vi "IdentifierResult.vi"(8 "error in (no error)":errorcluster, 11 "map":map{string, string}(c390)) -> (0 "error out":errorcluster, 2 "status":string, 3 "description":string)   [LabVIEW 2021]
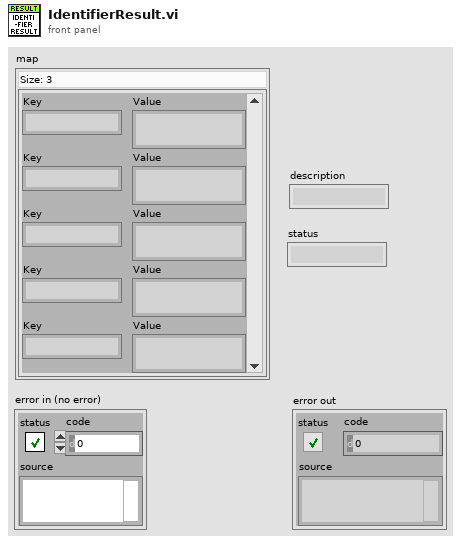
[diagram p1: front panel]
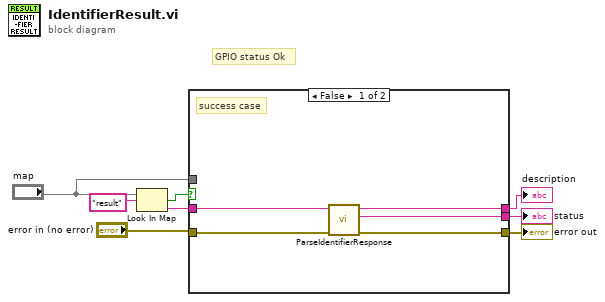
[diagram p0: block diagram]
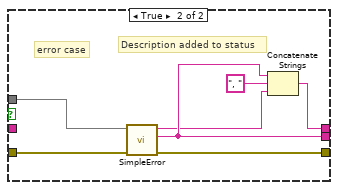
[diagram p2: hidden frame]
diagram:
  # "GPIO status Ok"
  n1 = Look In Map(map="map", key="result") -> (key not found?=w6:bool, value=w7:string)  [unwired: 1 in]
  n2 = case shown="False" w6 {
    tunnel: w7 -> [w13 _]
    tunnel: "error in (no error)" -> [w12 w20]
    tunnel: [w11 w19] -> w4
    tunnel: "map" -> [_ w18]
    tunnel: [w9 w14] -> w1
    tunnel: [w10 w16] -> w2
    frame False {
      # "success case"
      n3 = call "ParseIdentifierResponse.vi"("error in (no error)"=w12, "Value"=w13) -> ("error out"=w11:errorcluster, "status"=w10:string, "description"=w9:string)  [unwired: 7 in]
    }
    frame True {
      # "Description added to status"
      # "error case"
      n4 = call "SimpleError.vi"("error in (no error)"=w20, "map"=w18) -> ("error out"=w19:errorcluster, "status"=w16:string, "description"=w15:string)  [unwired: 7 in]
      n5 = Concatenate Strings(w16, ", " ("string"), w15) -> (w14:string)
    }
  }
  "error out" <- w4
  "status" <- w2
  "description" <- w1
